vi "U2 Reto.vi"() -> ()   [LabVIEW 2022 SP3]
uses:
  <vilib>/MakerHub/LINX/Public/Peripherals/Digital/Digital Read N Chans.vi
  <vilib>/MakerHub/LINX/Private/Local IO/LinxDigitalRead.vi
  <vilib>/MakerHub/LINX/Public/Utilities/Check Channel.vi
  <vilib>/MakerHub/LINX/Private/Utilties/Generate Error.vi
  <vilib>/MakerHub/LINX/Private/Device/Peripheral/Digital/Digital Read.vi
  <vilib>/MakerHub/LINX/Public/Utilities/Open Serial.vi
  <vilib>/MakerHub/LINX/LMH-LINX.lvlib
panel:
  in  "Serial Port":refnum<visa-resource-name>
  in  "rst":bool
  in  "RESET":bool
  in  "B2":bool
  in  "UP":bool
  in  "stop":bool
  out "Cuenta":u8
  in  "s/s":bool
  in  "START / STOP":bool
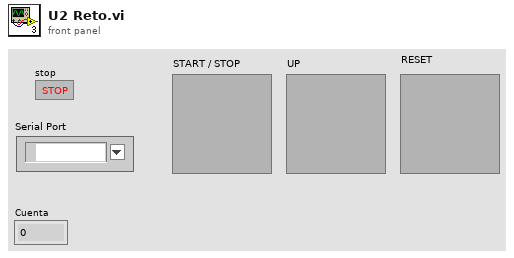
[diagram p1: front panel]
types:
  T1 = typedef "LMH-LINX.lvlib/LINX Ref.ctl" = cluster{"IO":T2, "Interface":T3, "LINX Device Config":T4}
  T2 = typedef "LMH-LINX.lvlib/Platform.ctl" = enum16{"Remote", "Local"}
  T3 = typedef "LMH-LINX.lvlib/Interface.ctl" = enum16{"Serial", "TCP"}
  T4 = typedef "LMH-LINX.lvlib/Device.lvlib/LINX Device Config.ctl" = cluster{"Interface":T3, "COM Port":refnum<visa-resource-name>, "TCP Configuration":T5, "Device Family":u8, "Device ID":u8, "Device Name":string, "TCP Ref":refnum<k5>, "Channels":T6}
  T5 = typedef "LMH-LINX.lvlib/Device.lvlib/TCP Config.ctl" = cluster{"IP Address":string, "Port":u16}
  T6 = typedef "LMH-LINX.lvlib/Channels.ctl" = cluster{"DI":u8[], "DO":u8[], "AI":u8[], "AO":u8[], "PWM":u8[], "QE":u8[], "UART":u8[], "I2C 2":u8[], "SPI":u8[], "CAN":u8[], "Servo":u8[], "AI Ref (V)":dbl, "AI Resolution (Bits)":u8, "AO Ref (V)":dbl, "AO Resolution (Bits)":u8}
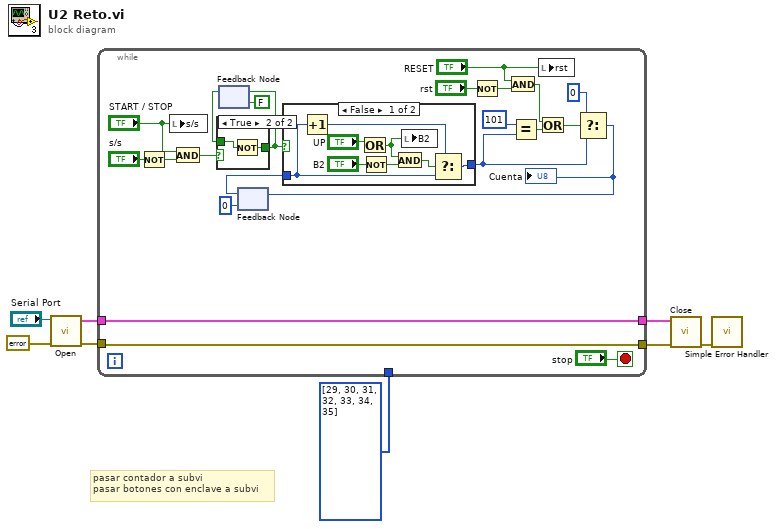
[diagram p0: block diagram]
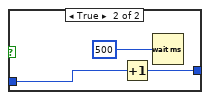
[diagram p3: hidden frame]
diagram:
  # "pasar contador a subvi\npasar botones con enclave a subvi"
  n1 = call-poly <vilib>:"Open.vi"("Error In"=errorcluster {"status"=FALSE, "code"=0, "source"=""}, "Serial Port"="Serial Port") -> ("Error Out"=w4:errorcluster, "LINX Resource"=w6:T1)  [unwired: 7 in, 1 out]
  n2 = while {
    tunnel: w6 -> [w10]
    tunnel: w4 -> [w9]
    tunnel: u8[] [29, 30, 31, 32, 33, 34, 35] ("Channels") -> [_]
    tunnel: [w10] -> w2
    tunnel: [w9] -> w1
    stop <- "stop" stop-if-true
    n3 = Not(x="s/s") -> (.not. x?=w30:bool)
    n4 = local write "s/s"("START / STOP") -> ()
    n5 = And(x="START / STOP", y=w30) -> (x .and. y?=w25:bool)
    n6 = feedback #1(FALSE) -> (w24:bool)
    n7 = case shown="True" w25 {
      tunnel: [w31 w33] -> w23
      tunnel: w24 -> [w31 w32]
      frame False {
      }
      frame True {
        n8 = Not(x=w32) -> (.not. x?=w33:bool)
      }
    }
    n9 = feedback-in #1(w23) -> ()
    n10 = feedback #2(u8 0) -> (w28:u8)
    n11 = case shown="False" w23 {
      tunnel: [w40 w42] -> w11
      tunnel: w28 -> [w34 w43]
      frame False {
        n12 = Increment(x=w34) -> (x+1=w41:u8)
        n13 = Or(x="UP") -> (x .or. y?=w35:bool)  [unwired: 1 in]
        n14 = Not(x="B2") -> (.not. x?=w38:bool)
        n15 = And(x=w35, y=w38) -> (x .and. y?=w37:bool)
        n16 = local write "B2"(w35) -> ()
        n17 = Select(t=w41, s=w37, f=w34) -> (s? t:f=w40:u8)
      }
      frame True {
        n18 = Increment(x=w43) -> (x+1=w42:u8)
        n19 = Wait (ms)(milliseconds to wait=u32 500) -> ()  [unwired: 1 out]
      }
    }
    n20 = Not(x="rst") -> (.not. x?=w17:bool)
    n21 = And(x="RESET", y=w17) -> (x .and. y?=w16:bool)
    n22 = Equal?(x=u8 101, y=w11) -> (x = y?=w20:bool)
    n23 = Or(x=w16, y=w20) -> (x .or. y?=w19:bool)
    n24 = local write "rst"("RESET") -> ()
    n25 = Select(t=u8 0, s=w19, f=w11) -> (s? t:f=w15:u8)
    "Cuenta" <- w15
    n26 = feedback-in #2(w15) -> ()
  }
  n27 = call <vilib>:"Close.vi"("Error In"=w1, "LINX Resource"=w2) -> ("Error Out"=w5:errorcluster)  [unwired: 9 in]
  n28 = call <vilib>:"Simple Error Handler.vi"("error in (no error)"=w5) -> ()  [unwired: 4 in, 5 out]
